vi "Get Scaling Coefficients.vi"(0 "device session in":refnum<class "Device Session.lvclass">, 11 "error in":errorcluster) -> (4 "device session out":refnum<class "Device Session.lvclass">, 6 "scaling coefficients":T1[](array[typedef]), 15 "error out":errorcluster)   [LabVIEW 2021, in "Device Session.lvclass"]
doc: "Returns the gain and offset values that you can use to scale data. This VI returns the scaling coefficients for each channel specified in the <B>channels to store</B> parameter of the <B>Configure Acquisition</B> VI. You must run the <B>Configure Acquisition</B> VI before running this VI.\n\n<B>Input Parameters</B>\n\n<B>device session in</B> is a reference to the Device Session object, which contains a session to each instrument design library used in this sample project. This parameter is obtained from the 'Open Session' VI.\n\n<B>error in</B> describes error conditions that occur before this node runs. This input provides standard 'error in' functionality.\n\n<B>Output Parameters</B>\n\n<B>device session out</B> passes a reference to the session to the next VI.\n\n<B>scaling coefficients</B> contains the scaling coefficients.\n\n<B>scaling coefficients.gain</B> is the gain coefficient.\n\n<B>scaling coefficients.offset</B> is the offset coefficient.\n\n<B>error out</B> contains error information. This output provides standard 'error out' functionality."
uses:
  Device Session.lvclass
  <instrlib>/_niInstr/Multirecord Acquisition/Interface/v1/Host/Public/Scaling Coefficient.ctl
  Device Session.lvclass/Device Session.ctl
  <instrlib>/_niInstr/Multirecord Acquisition/Interface/v1/Host/niInstr Multirecord Acquisition v1 Host.lvclass
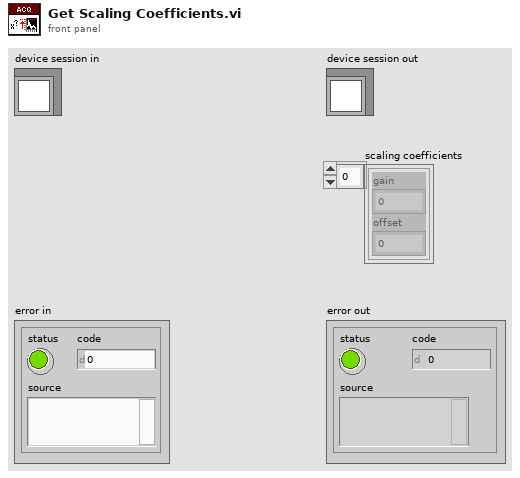
[diagram p1: front panel]
types:
  T1 = typedef "niInstr Multirecord Acquisition v1 Host.lvclass/Scaling Coefficient.ctl" = cluster{"gain":dbl, "offset":dbl}
  T2 = typedef "Device Session.lvclass/Device Session Object.ctl" = cluster{"fpga reference":T3, "reg bus":refnum<class "niInstr FIFO Register Bus v1 Host.lvclass">, "subsystem map":refnum<class "niInstr Subsystem Map v1 Host.lvclass">, "cal data":refnum<class "niHSAI Cal Data v1 Host.lvclass">, "config":refnum<class "niHSAI Group A Config v1 Host.lvclass">, "acquisition":refnum<class "niInstr Multirecord Acquisition v1 Host.lvclass">, "number of selected acq channels":u8, "selected acq channels":bool[], "number of channels":u32, "configured channels":bool[], "acq configuration":cluster{"number of samples":u64, "number of records":u64, "pretrigger samples":u64}, "actual channel configuration":T4[], "sample clock rate (Hz)":dbl, "scaling coefficients":T1[]}
  T3 = typedef "Device Session.lvclass/FPGA Refnum.ctl" = refnum<k20>
  T4 = typedef "niHSAI Types v1 Host.lvlib/Channel Configuration.ctl" = cluster{"channel":u32, "coupling":T5, "impedance":T6, "bandwidth":T7, "vertical range":dbl, "vertical offset":dbl}
  T5 = typedef "niHSAI Types v1 Host.lvlib/Coupling.ctl" = enum8{"Default", "DC", "AC"}
  T6 = typedef "niHSAI Types v1 Host.lvlib/Impedance.ctl" = enum8{"Default", "1 mega ohm", "50 ohm"}
  T7 = typedef "niHSAI Types v1 Host.lvlib/Bandwidth.ctl" = enum8{"Default", "Full Bandwidth", "Anti-alias Filter", "150 MHz"}
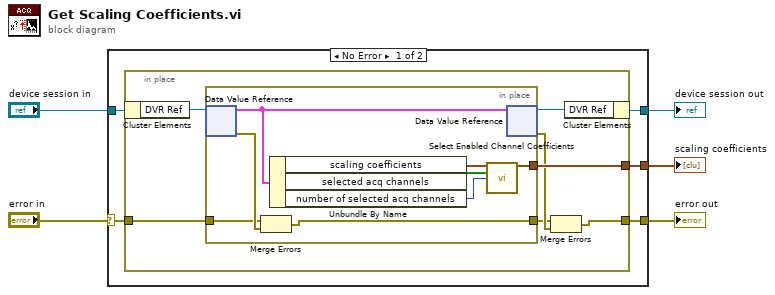
[diagram p0: block diagram]
diagram:
  n1 = case shown="No Error" "error in" {
    selector: "error in" -> [w10 w27]
    tunnel: "device session in" -> [w7 w26]
    tunnel: [w6 w26] -> w3
    tunnel: [w8 w27] -> w2
    tunnel: [w9 _] -> w1
    frame No Error {
      n2 = in-place {
        in-place-border: w10 -> [w17]
        in-place-border: [w16] -> w9
        in-place-border: [w13] -> w8
        n3 = in-place-cluster #1(w7) -> ("DVR Ref"=w12:refnum<data-value>)
        n4 = in-place {
          in-place-border: w17 -> [w23]
          in-place-border: [w18] -> w14
          in-place-border: [w22] -> w16
          n5 = in-place-dvr #2(w12) -> (w25:T2, w24:errorcluster)
          n6 = Merge Errors(w23, w24) -> (w18:errorcluster)
          n7 = Unbundle By Name(w25) -> ("scaling coefficients"=w21:T1[], "selected acq channels"=w20:bool[], "number of selected acq channels"=w19:u8)
          n8 = call "Select Enabled Channel Coefficients.vi"("configured scaling coefficients"=w21, "selected acq channels to store"=w20, "number of selected acq channels to store"=w19) -> ("stored scaling coefficients"=w22:T1[])  [unwired: 12 in]
          n9 = in-place-dvr #2(w25) -> (w11:refnum<data-value>, w15:errorcluster)
        }
        n10 = Merge Errors(w14, w15) -> (w13:errorcluster)
        n11 = in-place-cluster #1("DVR Ref"=w11) -> (w6:refnum<class "Device Session.lvclass">)
      }
    }
    frame Error {
    }
  }
  "error out" <- w2
  "device session out" <- w3
  "scaling coefficients" <- w1
